vi "MotorPositionControllerStart.vi"(0 "Device Info":T2={"Serial Number"=-1, "Channel"=0, "Port"=0}, 1 "Engaged":bool=TRUE, 5 "MotorPosCtrl Init Data":T1={"Rescale Factor"=1.0, "Velocity Limit"=20000.0, "Acceleration"=10000.0, "Kp"=2000.0, "Ki"=5.0, "Kd"=25000.0, "DeadBand"=0.0}, 11 "error in (no error)":errorcluster, 12 "Connection":u16(ring) items=["No Preference", "Remote", "Local"], 13 "Timeout (mSec)":i32=5000) -> (4 "Phidget ID":u64, 6 "Serial Number Return":i32, 10 "Attached?":bool, 15 "error out":errorcluster)   [LabVIEW 2020, in "Phidget Motor Position Controller.lvlib"]
doc: "${MotorPositionController:StartHeader}"
uses:
  <instrlib>/Phidgets/Phidget Motor Position Controller/Phidget Motor Position Controller.lvlib
panel:
  # "The default Velocity Limit and Acceleration settings seen here are not compatible with the DCC1100 BLDC Motor controller. They may both be set  to 200 (or some other compatible value) for the device to work."
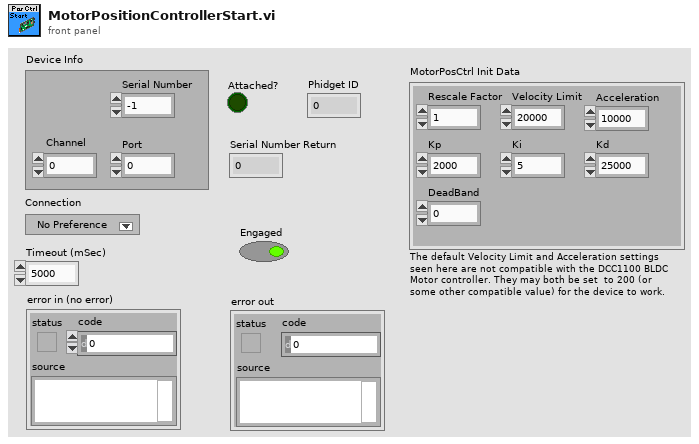
[diagram p1: front panel]
types:
  T1 = cluster{"Rescale Factor":dbl, "Velocity Limit":dbl, "Acceleration":dbl, "Kp":dbl, "Ki":dbl, "Kd":dbl, "DeadBand":dbl}
  T2 = cluster{"Serial Number":i32, "Channel":i32, "Port":i32}
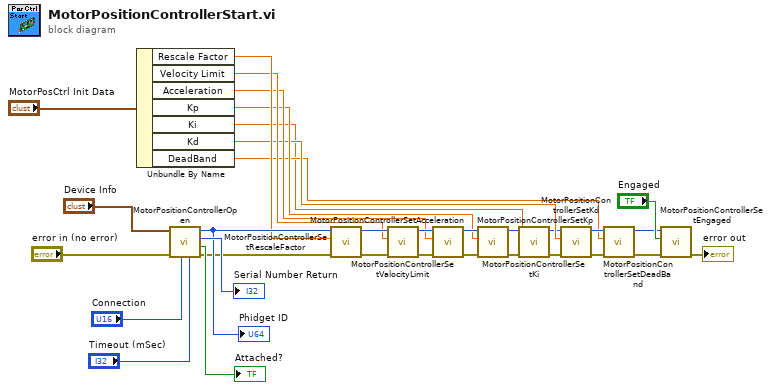
[diagram p0: block diagram]
diagram:
  n1 = Unbundle By Name("MotorPosCtrl Init Data") -> ("Rescale Factor"=w23:dbl, "Velocity Limit"=w20:dbl, "Acceleration"=w17:dbl, "Kp"=w12:dbl, "Ki"=w3:dbl, "Kd"=w11:dbl, "DeadBand"=w10:dbl)
  n2 = call <instrlib>:"MotorPositionControllerOpen.vi"("Timeout (mSec)"="Timeout (mSec)", "Connection"="Connection", "error in"="error in (no error)", "Device Info"="Device Info") -> ("error out"=w24:errorcluster, "Attached?"=→"Attached?":bool, "Serial Number Return"=→"Serial Number Return":i32, "Phidget ID"=w25:u64)  [unwired: 4 in]
  "Phidget ID" <- w25
  n3 = call <instrlib>:"MotorPositionControllerSetRescaleFactor.vi"("error in (no error)"=w24, "Rescale Factor"=w23, "Device In"=w25) -> ("error out"=w21:errorcluster, "Device Out"=w22:u64)  [unwired: 6 in]
  n4 = call <instrlib>:"MotorPositionControllerSetValocityLimit.vi"("error in (no error)"=w21, "Velocity Limit"=w20, "Device In"=w22) -> ("error out"=w18:errorcluster, "Device Out"=w19:u64)  [unwired: 6 in]
  n5 = call <instrlib>:"MotorPositionControllerSetAcceleration.vi"("error in (no error)"=w18, "Acceleration"=w17, "Device In"=w19) -> ("error out"=w15:errorcluster, "Device Out"=w16:u64)  [unwired: 6 in]
  n6 = call <instrlib>:"MotorPositionControllerSetKp.vi"("error in (no error)"=w15, "Kp"=w12, "Device In"=w16) -> ("error out"=w4:errorcluster, "Device Out"=w5:u64)  [unwired: 6 in]
  n7 = call <instrlib>:"MotorPositionControllerSetKi.vi"("error in (no error)"=w4, "Ki"=w3, "Device In"=w5) -> ("error out"=w7:errorcluster, "Device Out"=w6:u64)  [unwired: 6 in]
  n8 = call <instrlib>:"MotorPositionControllerSetKd.vi"("error in (no error)"=w7, "Kd"=w11, "Device In"=w6) -> ("error out"=w14:errorcluster, "Device Out"=w13:u64)  [unwired: 6 in]
  n9 = call <instrlib>:"MotorPositionControllerSetDeadBand.vi"("error in (no error)"=w14, "DeadBand"=w10, "Device In"=w13) -> ("error out"=w1:errorcluster, "Device Out"=w2:u64)  [unwired: 6 in]
  n10 = call <instrlib>:"MotorPositionControllerSetEngaged.vi"("error in (no error)"=w1, "Engaged"="Engaged", "Device In"=w2) -> ("error out"=→"error out":errorcluster)  [unwired: 6 in, 1 out]
